vi "Autonomous Independent.vi"() -> ()   [LabVIEW 2014]
doc: "This VI is called when autonomous begins, and will automatically be terminated when autonomous ends. You can carry out timed or sensor driven robot movement independently without needing to return to the caller."
uses:
  Control 1.ctl
  <vilib>/Rock Robotics/WPI/RobotDrive/WPI_RobotDriveGetSetRefNum.vi
  Robot Global Data.vi
  <vilib>/Rock Robotics/WPI/RobotDrive/WPI_RobotDriveArcadeDrive_Standard(NoSaturation).vi
  <vilib>/addons/control/pid/pid.llb/PID (DBL).vi
  <vilib>/addons/control/pid/NI_PID_pid.lvlib
panel:
  out "Distance":dbl
  # "Be sure to right-click and choose Data Operations>>Make Current Value default if you want to save the array values with the VI"
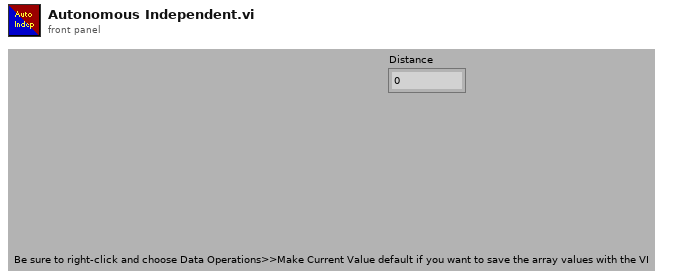
[diagram p1: front panel]
types:
  T1 = typedef "Control 1.ctl" = enum16{"initialize", "raise arms", "close arms", "raise #2", "rotate 90", "rotate 90 gyro", "forward", "stop"}
  T2 = typedef "WPI_GyroDevRef.ctl" = cluster{"DevStatus":errorcluster, "Analog Module":T3, "Analog Channel":T4, "Offset":dbl, "Gain (VoltsPerDegree/Second)":dbl}
  T3 = typedef "FPGA_TypedefAnalogModule.ctl" = enum16{"Controller 1"}
  T4 = typedef "FPGA_AIChannel.ctl" = enum8{"AI 0", "AI 1", "AI 2", "AI 3", "AI MXP 0", "AI MXP 1", "AI MXP 2", "AI MXP 3", "Invalid"}
  T5 = typedef "WPI_RobotDriveDevRef.ctl" = cluster{"DevStatus":errorcluster, "Motors[]":T6[], "Square Inputs":bool, "Max Output":dbl}
  T6 = typedef "WPI_MotorControlDeviceRef.ctl" = cluster{"DeviceStatus":errorcluster, "Type":T7, "PWM":cluster{"Controller":T8, "PWM Channel":T9, "DeadBand":T10}, "CAN":cluster{"Device Number":u8, "Control Mode":T11, "Semaphore":T12, "Max Vout":dbl, "TalonSRX Control Mode":T13}, "Invert":bool, "TransformRef":T14, "InvTransformRef":T14}
  T7 = typedef "WPI_MotorControlType.ctl" = enum16{"PWM", "CAN", "CANTalonSRX"}
  T8 = typedef "FPGA_TypedefDigitalModule.ctl" = enum16{"Controller 1"}
  T9 = typedef "FPGA_DIOPWMChannel.ctl" = enum8{"PWM 0", "PWM 1", "PWM 2", "PWM 3", "PWM 4", "PWM 5", "PWM 6", "PWM 7", "PWM 8", "PWM 9", "PWM MXP 0", "PWM MXP 1", "PWM MXP 2", "PWM MXP 3", "PWM MXP 4", "PWM MXP 5", "PWM MXP 6", "PWM MXP 7", "PWM MXP 8", "PWM MXP 9", "Invalid"}
  T10 = typedef "WPI_PWMDeadband.ctl" = cluster{"Name":string, "maxPositivePwm":i32, "minPositivePwm":i32, "centerPwm":i32, "maxNegativePwm":i32, "minNegativePwm":i32, "angularRange":u16}
  T11 = typedef "WPI_CANJaguar_ControlMode.ctl" = enum8{"Percent VBus", "Current", "Speed", "Position", "Voltage"}
  T12 = typedef "Semaphore RefNum" = refnum<k1>
  T13 = typedef "WPI_CANTalonSRX_APIControlMode.ctl" = enum8{"Percent VBus", "Speed", "Position", "Slave", "Unchanged / Invalid"}
  T14 = typedef "WPI_PWMTransform_ConPane.ctl" = refnum<vi>
  T15 = typedef "WPI_EncoderDevRef.ctl" = cluster{"DevStatus":errorcluster, "EncoderIndex":T16, "CounterIndex":T17, "DistancePerCount":dbl, "Decoding Type":T18}
  T16 = typedef "FPGA_EncoderIdx.ctl" = enum8{"Enc 0", "Enc 1", "Enc 2", "Enc 3", "Enc 4", "Enc 5", "Enc 6", "Enc 7", "Invalid"}
  T17 = typedef "FPGA_CounterCtrSystemIndex.ctl" = enum8{"Ctr 0", "Ctr 1", "Ctr 2", "Ctr 3", "Ctr 4", "Ctr 5", "Ctr 6", "Ctr 7", "Invalid"}
  T18 = typedef "WPI_EncoderType.ctl" = enum16{"1x", "2x", "4x"}
  T19 = cluster{"proportional gain (Kc)":dbl, "integral time (Ti, min)":dbl, "derivative time (Td, min)":dbl}
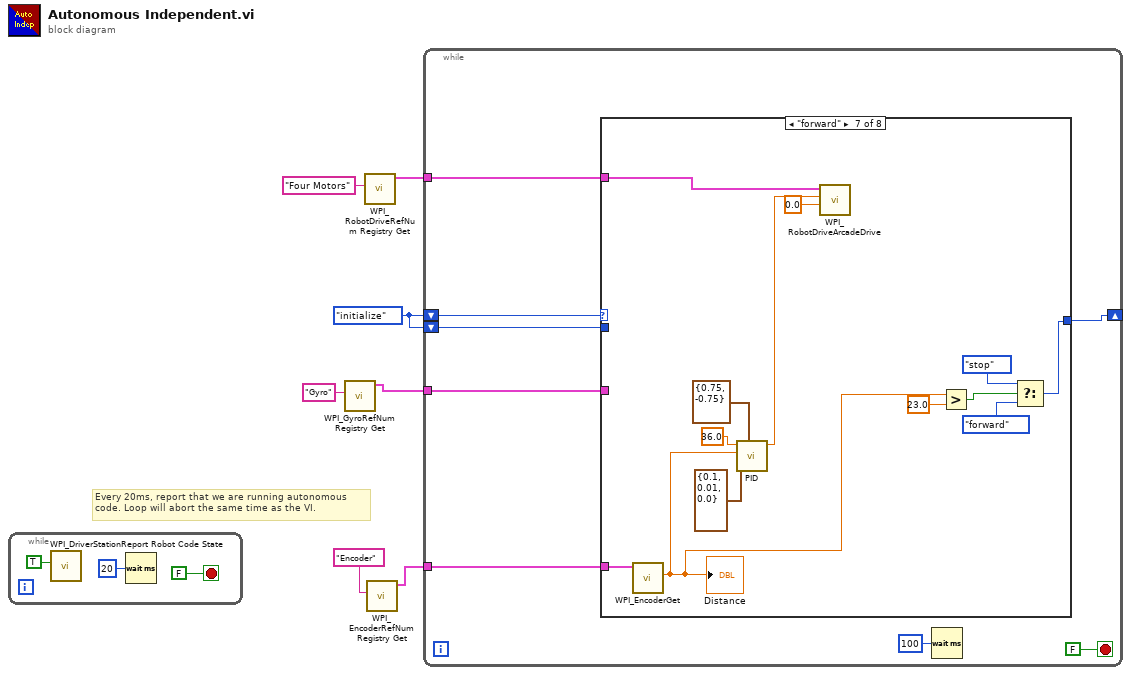
[diagram p0: block diagram]
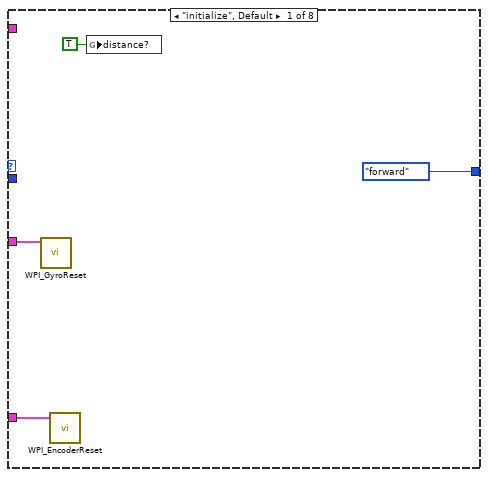
[diagram p2: hidden frame]
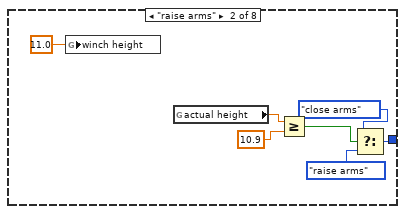
[diagram p3: hidden frame]
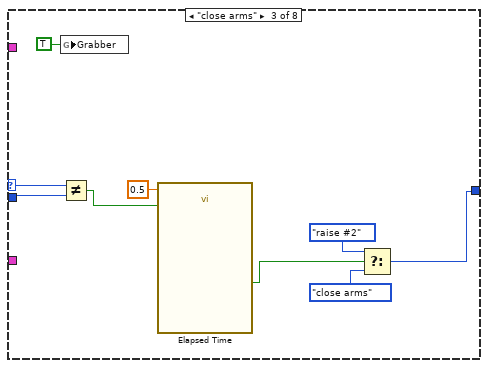
[diagram p4: hidden frame]
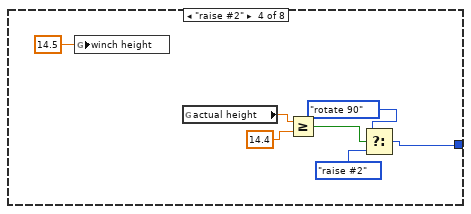
[diagram p5: hidden frame]
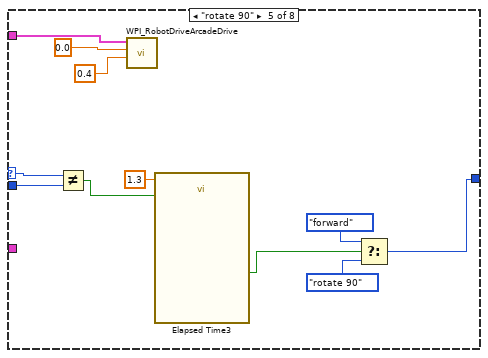
[diagram p6: hidden frame]
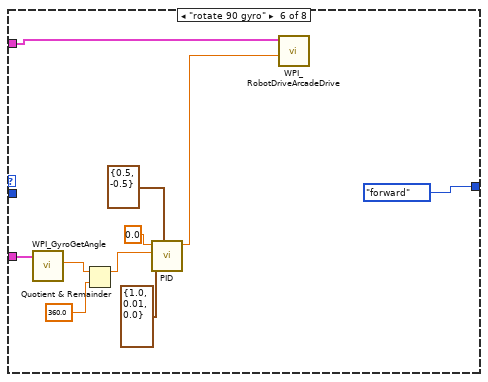
[diagram p7: hidden frame]
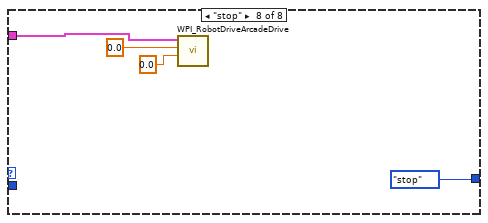
[diagram p8: hidden frame]
diagram:
  w6 = Control_1."initialize"
  # "Every 20ms, report that we are running autonomous\ncode. Loop will abort the same time as the VI."
  n1 = while {
    stop <- FALSE stop-if-true
    n2 = call <vilib>:"WPI_DriverStationReport Robot Code State.vi"("Autonomous"=TRUE) -> ()  [unwired: 10 in, 1 out]
    n3 = Wait (ms)(milliseconds to wait=u32 20) -> ()  [unwired: 1 out]
  }
  n4 = call <vilib>:"WPI_GyroRefNum Registry Get.vi"("refnum name"="Gyro") -> ("GyroDevRef"=w3:T2)  [unwired: 9 in, 1 out]
  n5 = call <vilib>:"WPI_RobotDriveRefNum Registry Get.vi"("refnum name"="Four Motors") -> ("RobotDriveDevRef"=w5:T5)  [unwired: 9 in, 1 out]
  n6 = call <vilib>:"WPI_EncoderRefNum Registry Get.vi"("refnum name"="Encoder") -> ("EncoderDevRef"=w1:T15)  [unwired: 9 in, 1 out]
  n7 = while {
    shift-right: [w16] -> _
    shift-left: w6 -> [w17]
    shift-left: w6 -> [w14]
    tunnel: w5 -> [w13]
    tunnel: w3 -> [w12]
    tunnel: w1 -> [w11]
    stop <- FALSE stop-if-true
    n8 = case shown="\"forward\"" w17 {
      selector: w17 -> [_ _ w31 _ w53 _ _ _]
      tunnel: [Control_1."forward" w27 w30 w40 w48 Control_1."forward" w77 Control_1."stop"] -> w16
      tunnel: w14 -> [_ _ w32 _ w54 _ _ _]
      tunnel: w13 -> [_ _ _ _ w47 w61 w76 w81]
      tunnel: w12 -> [w20 _ _ _ _ w66 _ _]
      tunnel: w11 -> [w19 _ _ _ _ _ w75 _]
      frame "initialize", Default {
        n9 = call <vilib>:"WPI_GyroReset.vi"("GyroDevRef"=w20) -> ()  [unwired: 9 in, 2 out]
        n10 = call <vilib>:"WPI_EncoderReset.vi"("EncoderDevRef"=w19) -> ()  [unwired: 9 in, 2 out]
        n11 = global write "Robot Global Data.vi" "distance?"(TRUE ("distance?")) -> ()
      }
      frame "raise arms" {
        n12 = global write "Robot Global Data.vi" "winch height"(11.0 ("winch height")) -> ()
        n13 = global read "Robot Global Data.vi" "actual height"() -> (w28:dbl)
        n14 = Greater Or Equal?(x=w28, y=10.9) -> (x >= y?=w25:bool)
        n15 = Select(t=Control_1."close arms", s=w25, f=Control_1."raise arms") -> (s? t:f=w27:T1)
      }
      frame "close arms" {
        n16 = global write "Robot Global Data.vi" "Grabber"(TRUE ("Grabber")) -> ()
        n17 = Not Equal?(x=w31, y=w32) -> (x != y?=w36:bool)
        n18 = call "Elapsed Time"("Time Target (s)"=0.5, "Reset"=w36) -> ("Time has Elapsed"=w35:bool)  [unwired: 10 in, 7 out]
        n19 = Select(t=Control_1."raise #2", s=w35, f=Control_1."close arms") -> (s? t:f=w30:T1)
      }
      frame "raise #2" {
        n20 = global write "Robot Global Data.vi" "winch height"(14.5 ("winch height")) -> ()
        n21 = global read "Robot Global Data.vi" "actual height"() -> (w44:dbl)
        n22 = Greater Or Equal?(x=w44, y=14.4) -> (x >= y?=w42:bool)
        n23 = Select(t=Control_1."rotate 90", s=w42, f=Control_1."raise #2") -> (s? t:f=w40:T1)
      }
      frame "rotate 90" {
        n24 = Not Equal?(x=w53, y=w54) -> (x != y?=w52:bool)
        n25 = call-poly <vilib>:"WPI_RobotDriveArcadeDrive.vi"("Y axis value"=0.4, "X axis value"=0.0, "RobotDriveDevRef"=w47) -> ()  [unwired: 6 in, 3 out]
        n26 = call "Elapsed Time3"("Time Target (s)"=1.3, "Reset"=w52) -> ("Time has Elapsed"=w51:bool)  [unwired: 10 in, 7 out]
        n27 = Select(t=Control_1."forward", s=w51, f=Control_1."rotate 90") -> (s? t:f=w48:T1)
      }
      frame "rotate 90 gyro" {
        n28 = call <vilib>:"WPI_GyroGetAngle.vi"("GyroDevRef"=w66) -> ("Angle"=w65:dbl)  [unwired: 7 in, 3 out]
        n29 = Quotient & Remainder(x=w65, y=360.0) -> (x-y*floor(x/y)=w63:dbl)  [unwired: 1 out]
        n30 = call-poly <vilib>:"PID.vi"("output range"=cluster{"output high":dbl, "output low":dbl} {"output high"=0.5, "output low"=-0.5}, "PID gains"=T19 {"proportional gain (Kc)"=1.0, "integral time (Ti, min)"=0.01, "derivative time (Td, min)"=0.0}, "process variable"=w63, "setpoint"=0.0) -> ("output"=w60:dbl)  [unwired: 6 in, 1 out]
        n31 = call-poly <vilib>:"WPI_RobotDriveArcadeDrive.vi"("Y axis value"=w60, "RobotDriveDevRef"=w61) -> ()  [unwired: 7 in, 3 out]
      }
      frame "forward" {
        n32 = call <vilib>:"WPI_EncoderGet.vi"("EncoderDevRef"=w75) -> ("Distance"=w68:dbl)  [unwired: 5 in, 5 out]
        "Distance" <- w68
        n33 = call-poly <vilib>:"PID.vi"("output range"=cluster{"output high":dbl, "output low":dbl} {"output high"=0.75, "output low"=-0.75}, "PID gains"=T19 {"proportional gain (Kc)"=0.1, "integral time (Ti, min)"=0.01, "derivative time (Td, min)"=0.0}, "process variable"=w68, "setpoint"=36.0) -> ("output"=w71:dbl)  [unwired: 6 in, 1 out]
        n34 = call-poly <vilib>:"WPI_RobotDriveArcadeDrive.vi"("Y axis value"=0.0, "X axis value"=w71, "RobotDriveDevRef"=w76) -> ()  [unwired: 6 in, 3 out]
        n35 = Greater?(x=w68, y=23.0) -> (0:w69:bool)
        n36 = Select(t=Control_1."stop", s=w69, f=Control_1."forward") -> (s? t:f=w77:T1)
      }
      frame "stop" {
        n37 = call-poly <vilib>:"WPI_RobotDriveArcadeDrive.vi"("Y axis value"=0.0, "X axis value"=0.0, "RobotDriveDevRef"=w81) -> ()  [unwired: 6 in, 3 out]
      }
    }
    n38 = Wait (ms)(milliseconds to wait=u32 100) -> ()  [unwired: 1 out]
  }
